vi "Finish.vi"   [LabVIEW 2020]
doc: "This VIcloses device references, sends final commands to the network tables and the joysticks, and terminates all command and control loops."
uses:
  GlobalDrivebase.vi
  GlobalDriverStationCommands.vi
  GlobalArm.vi
  GlobalGripper.vi
  GlobalHopper.vi
types:
  T1 = typedef "WPI_SolenoidDevRef.ctl" = cluster{"DevStatus":errorcluster, "Pneumatics Control Module":u8, "Forward Solenoid Channel":T2, "Reverse Solenoid Channel":T2}
  T2 = typedef "WPI_SolenoidChannel.ctl" = enum8{"Solenoid 0", "Solenoid 1", "Solenoid 2", "Solenoid 3", "Solenoid 4", "Solenoid 5", "Solenoid 6", "Solenoid 7", "Solenoid 8", "Solenoid 9", "Solenoid 10", "Solenoid 11", "Solenoid 12", "Solenoid 13", "Solenoid 14", "Solenoid 15", "Invalid"}
  T3 = typedef "WPI_DigitalInputDevRef.ctl" = cluster{"DevStatus":errorcluster, "DIO Channel":T4}
  T4 = typedef "FPGA_DIOChannel.ctl" = enum8{"DIO 0", "DIO 1", "DIO 2", "DIO 3", "DIO 4", "DIO 5", "DIO 6", "DIO 7", "DIO 8", "DIO 9", "DIO MXP 0", "DIO MXP 1", "DIO MXP 2", "DIO MXP 3", "DIO MXP 4", "DIO MXP 5", "DIO MXP 6", "DIO MXP 7", "DIO MXP 8", "DIO MXP 9", "DIO MXP 10", "DIO MXP 11", "DIO MXP 12", "DIO MXP 13", "DIO MXP 14", "DIO MXP 15", "SPI Port CS1", "SPI Port CS2", "SPI Port CS3", "SPI Port MISO", "SPI Port MOSI", "Invalid"}
  T5 = typedef "Color Sensor V3 DevRef.ctl" = cluster{"I2CDevRef":T6}
  T6 = typedef "WPI_I2CDevRef.ctl" = cluster{"DevStatus":errorcluster, "Device Address":u8, "Handle":i32, "I2C Bus":T7}
  T7 = typedef "i2c_bus.ctl" = enum16{"I2C On-Board", "I2C MXP", "Invalid"}
  T8 = typedef "WPI_JoystickDevRef.ctl" = cluster{"Device":T9}
  T9 = typedef "WPI_JoystickDeviceEnum.ctl" = enum16{"USB 0", "USB 1", "USB 2", "USB 3", "USB 4", "USB 5"}
  T10 = typedef "WPI_MotorControlDeviceRef.ctl" = cluster{"DeviceStatus":errorcluster, "Type":T11, "PWM":cluster{"PWM Channel":T12, "DeadBand":T13}, "CAN":cluster{"Device Number":u8, "SetOutput VI Ref":variant, "GetOutput VI Ref":variant, "Enable VI Ref":variant, "Disable VI Ref":variant, "Data":variant}, "Invert":bool, "DIO PWM":cluster{"PWM \"Enable\" Channel":T12, "DIOChannel":T4, "PWM Rate":dbl}}
  T11 = typedef "WPI_MotorControlType.ctl" = enum16{"PWM", "CAN", "DIO PWM"}
  T12 = typedef "FPGA_DIOPWMChannel.ctl" = enum8{"PWM 0", "PWM 1", "PWM 2", "PWM 3", "PWM 4", "PWM 5", "PWM 6", "PWM 7", "PWM 8", "PWM 9", "PWM MXP 0", "PWM MXP 1", "PWM MXP 2", "PWM MXP 3", "PWM MXP 4", "PWM MXP 5", "PWM MXP 6", "PWM MXP 7", "PWM MXP 8", "PWM MXP 9", "Invalid"}
  T13 = typedef "WPI_PWMDeadband.ctl" = cluster{"Name":string, "maxPositivePwm":i32, "minPositivePwm":i32, "centerPwm":i32, "maxNegativePwm":i32, "minNegativePwm":i32, "angularRange":u16}
  T14 = typedef "WPI_PotentiometerDevRef.ctl" = cluster{"DevStatus":errorcluster, "Analog Channel":T15, "Invert Output":bool}
  T15 = typedef "FPGA_AIChannel.ctl" = enum8{"AI 0", "AI 1", "AI 2", "AI 3", "AI MXP 0", "AI MXP 1", "AI MXP 2", "AI MXP 3", "Invalid"}
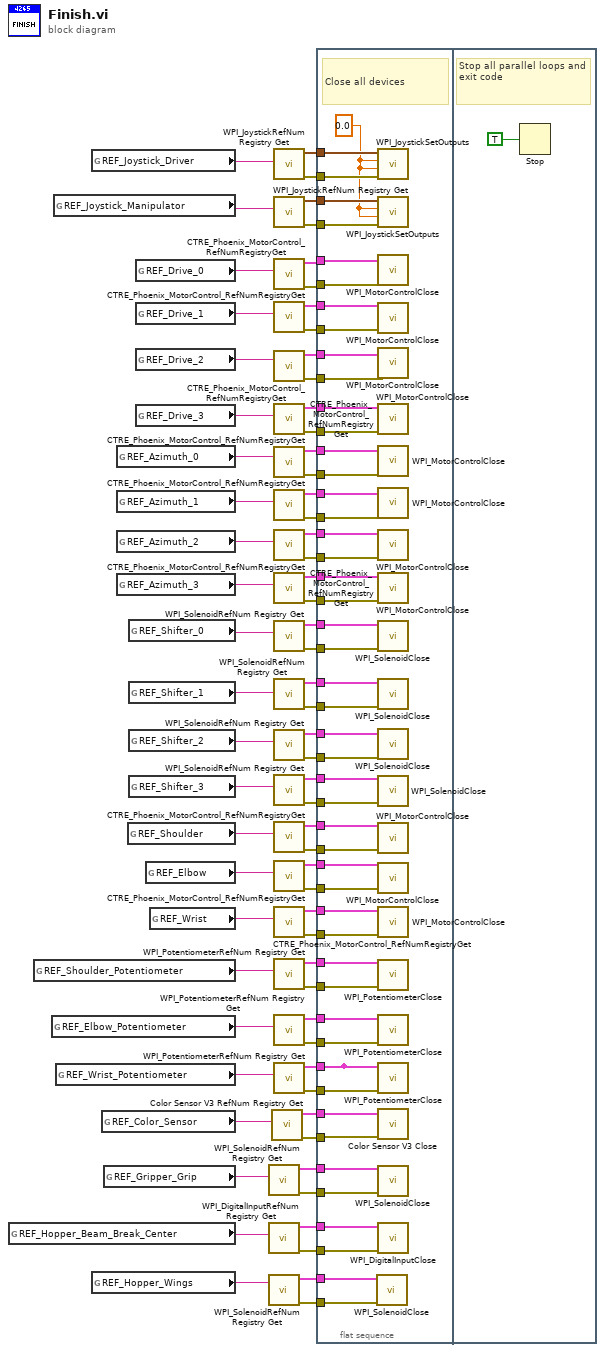
[diagram p0: block diagram]
diagram:
  n1 = global read "GlobalHopper.vi" "REF_Hopper_Beam_Break_Center"() -> (w6:string)
  n2 = global read "GlobalArm.vi" "REF_Shoulder_Potentiometer"() -> (w13:string)
  n3 = global read "GlobalArm.vi" "REF_Elbow_Potentiometer"() -> (w14:string)
  n4 = global read "GlobalDriverStationCommands.vi" "REF_Joystick_Manipulator"() -> (w31:string)
  n5 = global read "GlobalArm.vi" "REF_Wrist_Potentiometer"() -> (w15:string)
  n6 = global read "GlobalDriverStationCommands.vi" "REF_Joystick_Driver"() -> (w32:string)
  n7 = global read "GlobalHopper.vi" "REF_Hopper_Wings"() -> (w3:string)
  n8 = global read "GlobalGripper.vi" "REF_Color_Sensor"() -> (w12:string)
  n9 = global read "GlobalGripper.vi" "REF_Gripper_Grip"() -> (w7:string)
  n10 = global read "GlobalDrivebase.vi" "REF_Azimuth_0"() -> (w44:string)
  n11 = global read "GlobalDrivebase.vi" "REF_Azimuth_1"() -> (w43:string)
  n12 = global read "GlobalDrivebase.vi" "REF_Azimuth_2"() -> (w42:string)
  n13 = global read "GlobalDrivebase.vi" "REF_Azimuth_3"() -> (w41:string)
  n14 = global read "GlobalArm.vi" "REF_Shoulder"() -> (w23:string)
  n15 = global read "GlobalDrivebase.vi" "REF_Shifter_0"() -> (w36:string)
  n16 = global read "GlobalDrivebase.vi" "REF_Shifter_1"() -> (w35:string)
  n17 = global read "GlobalDrivebase.vi" "REF_Shifter_2"() -> (w34:string)
  n18 = global read "GlobalDrivebase.vi" "REF_Shifter_3"() -> (w33:string)
  n19 = global read "GlobalDrivebase.vi" "REF_Drive_0"() -> (w40:string)
  n20 = global read "GlobalDrivebase.vi" "REF_Drive_1"() -> (w39:string)
  n21 = global read "GlobalDrivebase.vi" "REF_Drive_2"() -> (w38:string)
  n22 = global read "GlobalDrivebase.vi" "REF_Drive_3"() -> (w37:string)
  n23 = global read "GlobalArm.vi" "REF_Elbow"() -> (w22:string)
  n24 = global read "GlobalArm.vi" "REF_Wrist"() -> (w24:string)
  n25 = call <vilib>:"WPI_SolenoidRefNum Registry Get.vi"("refnum name"=w7) -> ("error out"=w8:errorcluster, "SolenoidDevRef"=w9:T1)  [unwired: 9 in]
  n26 = call <vilib>:"WPI_DigitalInputRefNum Registry Get.vi"("refnum name"=w6) -> ("error out"=w4:errorcluster, "DigitalInputDevRef"=w5:T3)  [unwired: 9 in]
  n27 = call <vilib>:"WPI_SolenoidRefNum Registry Get.vi"("refnum name"=w3) -> ("error out"=w1:errorcluster, "SolenoidDevRef"=w2:T1)  [unwired: 9 in]
  n28 = call <vilib>:"Color Sensor V3 RefNum Registry Get.vi"("refnum name"=w12) -> ("error out"=w10:errorcluster, "ColorSensorDevRef"=w11:T5)  [unwired: 9 in]
  n29 = call <vilib>:"WPI_JoystickRefNum Registry Get.vi"("refnum name"=w32) -> ("error out"=w71:errorcluster, "JoystickDevRef"=w72:T8)  [unwired: 9 in]
  n30 = call <vilib>:"WPI_JoystickRefNum Registry Get.vi"("refnum name"=w31) -> ("error out"=w69:errorcluster, "JoystickDevRef"=w70:T8)  [unwired: 9 in]
  n31 = call <vilib>:"CTRE_Phoenix_MotorControl_RefNumRegistryGet.vi"("refnum name"=w40) -> ("error out"=w63:errorcluster, "PhoenixMotorControlDevRef"=w64:T10)  [unwired: 9 in]
  n32 = call <vilib>:"CTRE_Phoenix_MotorControl_RefNumRegistryGet.vi"("refnum name"=w39) -> ("error out"=w59:errorcluster, "PhoenixMotorControlDevRef"=w62:T10)  [unwired: 9 in]
  n33 = call <vilib>:"CTRE_Phoenix_MotorControl_RefNumRegistryGet.vi"("refnum name"=w38) -> ("error out"=w60:errorcluster, "PhoenixMotorControlDevRef"=w61:T10)  [unwired: 9 in]
  n34 = call <vilib>:"CTRE_Phoenix_MotorControl_RefNumRegistryGet.vi"("refnum name"=w37) -> ("error out"=w67:errorcluster, "PhoenixMotorControlDevRef"=w68:T10)  [unwired: 9 in]
  n35 = call <vilib>:"CTRE_Phoenix_MotorControl_RefNumRegistryGet.vi"("refnum name"=w44) -> ("error out"=w54:errorcluster, "PhoenixMotorControlDevRef"=w58:T10)  [unwired: 9 in]
  n36 = call <vilib>:"CTRE_Phoenix_MotorControl_RefNumRegistryGet.vi"("refnum name"=w43) -> ("error out"=w53:errorcluster, "PhoenixMotorControlDevRef"=w57:T10)  [unwired: 9 in]
  n37 = call <vilib>:"CTRE_Phoenix_MotorControl_RefNumRegistryGet.vi"("refnum name"=w42) -> ("error out"=w52:errorcluster, "PhoenixMotorControlDevRef"=w56:T10)  [unwired: 9 in]
  n38 = call <vilib>:"CTRE_Phoenix_MotorControl_RefNumRegistryGet.vi"("refnum name"=w41) -> ("error out"=w51:errorcluster, "PhoenixMotorControlDevRef"=w55:T10)  [unwired: 9 in]
  n39 = call <vilib>:"WPI_SolenoidRefNum Registry Get.vi"("refnum name"=w36) -> ("error out"=w49:errorcluster, "SolenoidDevRef"=w50:T1)  [unwired: 9 in]
  n40 = call <vilib>:"WPI_SolenoidRefNum Registry Get.vi"("refnum name"=w35) -> ("error out"=w47:errorcluster, "SolenoidDevRef"=w48:T1)  [unwired: 9 in]
  n41 = call <vilib>:"WPI_SolenoidRefNum Registry Get.vi"("refnum name"=w34) -> ("error out"=w45:errorcluster, "SolenoidDevRef"=w46:T1)  [unwired: 9 in]
  n42 = call <vilib>:"WPI_SolenoidRefNum Registry Get.vi"("refnum name"=w33) -> ("error out"=w65:errorcluster, "SolenoidDevRef"=w66:T1)  [unwired: 9 in]
  n43 = call <vilib>:"CTRE_Phoenix_MotorControl_RefNumRegistryGet.vi"("refnum name"=w23) -> ("error out"=w27:errorcluster, "PhoenixMotorControlDevRef"=w28:T10)  [unwired: 9 in]
  n44 = call <vilib>:"CTRE_Phoenix_MotorControl_RefNumRegistryGet.vi"("refnum name"=w22) -> ("error out"=w25:errorcluster, "PhoenixMotorControlDevRef"=w26:T10)  [unwired: 9 in]
  n45 = call <vilib>:"CTRE_Phoenix_MotorControl_RefNumRegistryGet.vi"("refnum name"=w24) -> ("error out"=w29:errorcluster, "PhoenixMotorControlDevRef"=w30:T10)  [unwired: 9 in]
  n46 = call <vilib>:"WPI_PotentiometerRefNum Registry Get.vi"("refnum name"=w13) -> ("error out"=w20:errorcluster, "PotDevRef"=w21:T14)  [unwired: 9 in]
  n47 = call <vilib>:"WPI_PotentiometerRefNum Registry Get.vi"("refnum name"=w14) -> ("error out"=w18:errorcluster, "PotDevRef"=w19:T14)  [unwired: 9 in]
  n48 = call <vilib>:"WPI_PotentiometerRefNum Registry Get.vi"("refnum name"=w15) -> ("error out"=w16:errorcluster, "PotDevRef"=w17:T14)  [unwired: 9 in]
  n49 = flat-sequence {
    tunnel: w64 -> [w121]
    tunnel: w62 -> [w120]
    tunnel: w63 -> [w119]
    tunnel: w72 -> [w118]
    tunnel: w71 -> [w117]
    tunnel: w70 -> [w116]
    tunnel: w69 -> [w115]
    tunnel: w68 -> [w113]
    tunnel: w67 -> [w112]
    tunnel: w66 -> [w111]
    tunnel: w65 -> [w110]
    tunnel: w61 -> [w109]
    tunnel: w60 -> [w108]
    tunnel: w59 -> [w107]
    tunnel: w58 -> [w106]
    tunnel: w57 -> [w105]
    tunnel: w56 -> [w104]
    tunnel: w55 -> [w103]
    tunnel: w54 -> [w102]
    tunnel: w53 -> [w101]
    tunnel: w52 -> [w100]
    tunnel: w51 -> [w99]
    tunnel: w50 -> [w98]
    tunnel: w49 -> [w97]
    tunnel: w48 -> [w96]
    tunnel: w47 -> [w95]
    tunnel: w46 -> [w94]
    tunnel: w45 -> [w93]
    tunnel: w30 -> [w92]
    tunnel: w29 -> [w91]
    tunnel: w28 -> [w90]
    tunnel: w27 -> [w89]
    tunnel: w26 -> [w88]
    tunnel: w25 -> [w87]
    tunnel: w21 -> [w86]
    tunnel: w20 -> [w85]
    tunnel: w19 -> [w84]
    tunnel: w18 -> [w83]
    tunnel: [w81] -> _
    tunnel: w16 -> [w82]
    tunnel: w17 -> [w81]
    tunnel: w11 -> [w80]
    tunnel: w10 -> [w79]
    tunnel: w9 -> [w78]
    tunnel: w8 -> [w77]
    tunnel: w5 -> [w76]
    tunnel: w4 -> [w75]
    tunnel: w2 -> [w74]
    tunnel: w1 -> [w73]
    frame #0 {
      w114 = sgl 0.0 ("Left Rumble")
      # "Close all devices"
      n50 = call <vilib>:"WPI_SolenoidClose.vi"("error in (no error)"=w73, "SolenoidDevRef"=w74) -> ()  [unwired: 9 in, 1 out]
      n51 = call <vilib>:"WPI_JoystickSetOutputs.vi"("error in (no error)"=w117, "Right Rumble"=w114, "Left Rumble"=w114, "JoystickDevRef"=w118) -> ()  [unwired: 6 in, 2 out]
      n52 = call <vilib>:"WPI_JoystickSetOutputs.vi"("error in (no error)"=w115, "Right Rumble"=w114, "Left Rumble"=w114, "JoystickDevRef"=w116) -> ()  [unwired: 6 in, 2 out]
      n53 = call <vilib>:"WPI_MotorControlClose.vi"("error in"=w119, "MotorControlDevRef"=w121) -> ()  [unwired: 9 in, 1 out]
      n54 = call <vilib>:"WPI_MotorControlClose.vi"("error in"=w107, "MotorControlDevRef"=w120) -> ()  [unwired: 9 in, 1 out]
      n55 = call <vilib>:"WPI_MotorControlClose.vi"("error in"=w108, "MotorControlDevRef"=w109) -> ()  [unwired: 9 in, 1 out]
      n56 = call <vilib>:"WPI_MotorControlClose.vi"("error in"=w112, "MotorControlDevRef"=w113) -> ()  [unwired: 9 in, 1 out]
      n57 = call <vilib>:"WPI_MotorControlClose.vi"("error in"=w102, "MotorControlDevRef"=w106) -> ()  [unwired: 9 in, 1 out]
      n58 = call <vilib>:"WPI_MotorControlClose.vi"("error in"=w101, "MotorControlDevRef"=w105) -> ()  [unwired: 9 in, 1 out]
      n59 = call <vilib>:"WPI_MotorControlClose.vi"("error in"=w100, "MotorControlDevRef"=w104) -> ()  [unwired: 9 in, 1 out]
      n60 = call <vilib>:"WPI_MotorControlClose.vi"("error in"=w99, "MotorControlDevRef"=w103) -> ()  [unwired: 9 in, 1 out]
      n61 = call <vilib>:"WPI_SolenoidClose.vi"("error in (no error)"=w97, "SolenoidDevRef"=w98) -> ()  [unwired: 9 in, 1 out]
      n62 = call <vilib>:"WPI_SolenoidClose.vi"("error in (no error)"=w95, "SolenoidDevRef"=w96) -> ()  [unwired: 9 in, 1 out]
      n63 = call <vilib>:"WPI_SolenoidClose.vi"("error in (no error)"=w93, "SolenoidDevRef"=w94) -> ()  [unwired: 9 in, 1 out]
      n64 = call <vilib>:"WPI_SolenoidClose.vi"("error in (no error)"=w110, "SolenoidDevRef"=w111) -> ()  [unwired: 9 in, 1 out]
      n65 = call <vilib>:"WPI_MotorControlClose.vi"("error in"=w89, "MotorControlDevRef"=w90) -> ()  [unwired: 9 in, 1 out]
      n66 = call <vilib>:"WPI_MotorControlClose.vi"("error in"=w87, "MotorControlDevRef"=w88) -> ()  [unwired: 9 in, 1 out]
      n67 = call <vilib>:"WPI_MotorControlClose.vi"("error in"=w91, "MotorControlDevRef"=w92) -> ()  [unwired: 9 in, 1 out]
      n68 = call <vilib>:"WPI_PotentiometerClose.vi"("error in"=w85, "PotDevRef"=w86) -> ()  [unwired: 9 in, 1 out]
      n69 = call <vilib>:"WPI_PotentiometerClose.vi"("error in"=w83, "PotDevRef"=w84) -> ()  [unwired: 9 in, 1 out]
      n70 = call <vilib>:"WPI_PotentiometerClose.vi"("error in"=w82, "PotDevRef"=w81) -> ()  [unwired: 9 in, 1 out]
      n71 = call <vilib>:"Color Sensor V3 Close.vi"("error in (no error)"=w79, "ColorSensorDevRef in"=w80) -> ()  [unwired: 9 in, 1 out]
      n72 = call <vilib>:"WPI_SolenoidClose.vi"("error in (no error)"=w77, "SolenoidDevRef"=w78) -> ()  [unwired: 9 in, 1 out]
      n73 = call <vilib>:"WPI_DigitalInputClose.vi"("error in (no error)"=w75, "DigitalInputDevRef"=w76) -> ()  [unwired: 9 in, 1 out]
    }
    frame #1 {
      # "Stop all parallel loops and exit code"
      n74 = Stop(stop? (T)=TRUE ("Quit")) -> ()
    }
  }
